vi "VMtoStr.vi"(3 "VariableManager in":refnum<class "VariableManager.lvclass">) -> (1 "VariablesString":string)   [LabVIEW 2013]
uses:
  VariableManager/VariableManager.lvclass
  Variable/Variable.lvclass
  SequenceIndex/SequenceIndex.lvclass
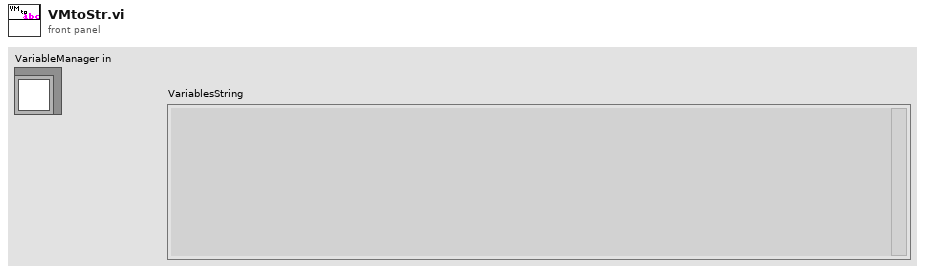
[diagram p1: front panel]
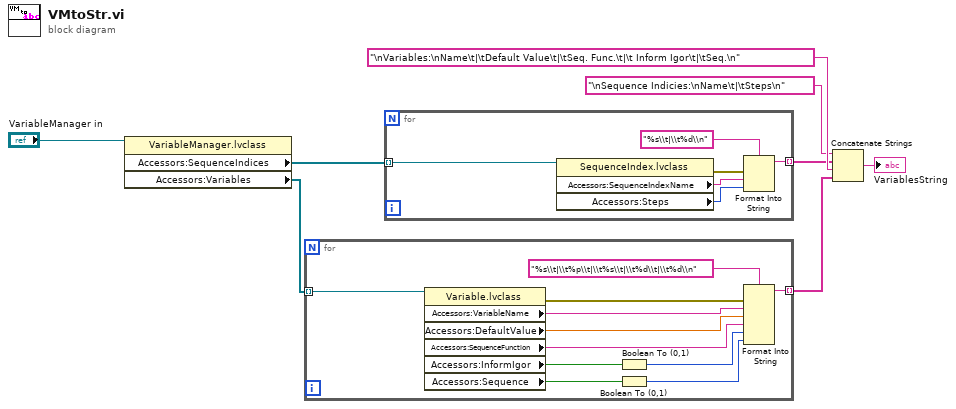
[diagram p0: block diagram]
diagram:
  n1 = property class="VariableManager.lvclass"(reference="VariableManager in") -> ("Accessors:SequenceIndices"=w7:refnum<class "SequenceIndex.lvclass">[], "Accessors:Variables"=w8:refnum<class "Variable.lvclass">[])  [unwired: 1 in, 2 out]
  n2 = for {
    tunnel: [w18] -> w5 mode=indexing
    tunnel: w8 -> [w15] mode=indexing
    n3 = property class="Variable.lvclass"(reference=w15) -> (error out=w9:errorcluster, "Accessors:VariableName"=w10:string, "Accessors:DefaultValue"=w11:dbl, "Accessors:SequenceFunction"=w12:string, "Accessors:InformIgor"=w13:bool, "Accessors:Sequence"=w14:bool)  [unwired: 1 in, 1 out]
    n4 = Boolean To (0,1)(Boolean=w13) -> (0, 1=w16:i16)
    n5 = Boolean To (0,1)(Boolean=w14) -> (0, 1=w17:i16)
    n6 = Format Into String(format string="%s\\t|\\t%p\\t|\\t%s\\t|\\t%d\\t|\\t%d\\n", error in=w9, w10, w11, w12, w16, w17) -> (resulting string=w18:string)  [unwired: 1 in, 1 out]
  }
  n7 = for {
    tunnel: w7 -> [w23] mode=indexing
    tunnel: [w24] -> w2 mode=indexing
    n8 = property class="SequenceIndex.lvclass"(reference=w23) -> (error out=w22:errorcluster, "Accessors:SequenceIndexName"=w21:string, "Accessors:Steps"=w20:u32)  [unwired: 1 in, 1 out]
    n9 = Format Into String(format string="%s\\t|\\t%d\\n", error in=w22, w21, w20) -> (resulting string=w24:string)  [unwired: 1 in, 1 out]
  }
  n10 = Concatenate Strings("\nSequence Indicies:\nName\t|\tSteps\n" ("string"), w2, "\nVariables:\nName\t|\tDefault Value\t|\tSeq. Func.\t|\t Inform Igor\t|\tSeq.\n" ("string"), w5) -> (→"VariablesString":string)
